vi "LIDAR Sensor Fusion 2.vi"() -> ()   [LabVIEW 2019]
panel:
  in  "Pointed at Target":bool
  out "Fused Range (in)":dbl
  in  "Estimate Range (in)":dbl
  in  "LIDAR Range (in)":dbl
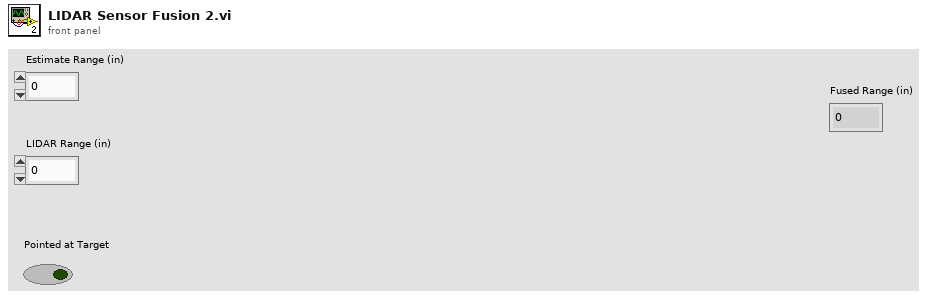
[diagram p1: front panel]
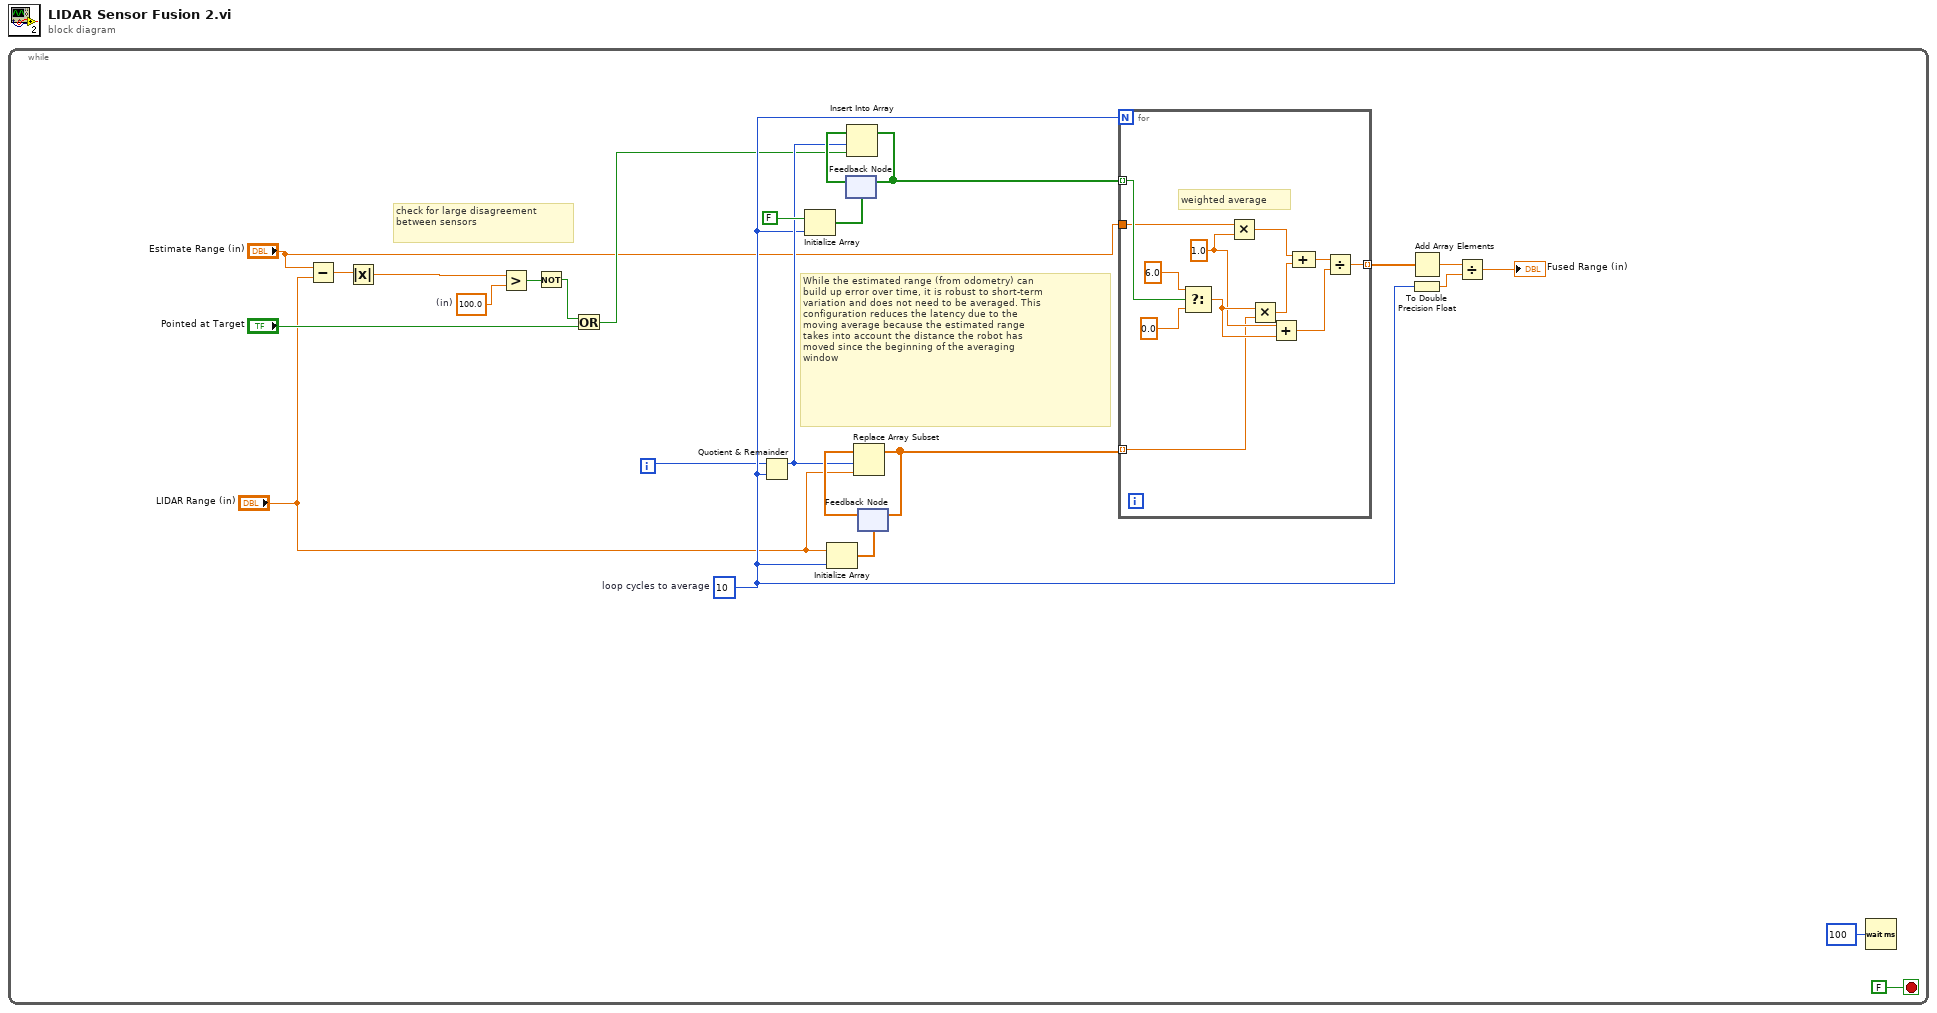
[diagram p0: block diagram]
diagram:
  n1 = while {
    i -> [w2]
    stop <- FALSE stop-if-true
    w6 = 10  # loop cycles to average
    w23 = 100.0  # (in)
    # "While the estimated range (from odometry) can \nbuild up error over time, it is robust to short-term\nvariation and does not need to be averaged. This\nconfiguration reduces the latency due to the \nmoving average because the estimated range\ntakes into account the distance the robot has\nmoved since the beginning of the averaging \nwindow"
    # "check for large disagreement\nbetween sensors"
    n2 = Subtract(x="Estimate Range (in)", y="LIDAR Range (in)") -> (x-y=w25:dbl)
    n3 = Absolute Value(x=w25) -> (abs(x)=w24:dbl)
    n4 = Greater?(x=w24, y=w23) -> (0:w22:bool)
    n5 = Not(x=w22) -> (.not. x?=w21:bool)
    n6 = Or(x=w21, y="Pointed at Target") -> (x .or. y?=w4:bool)
    n7 = Quotient & Remainder(x=w2, y=w6) -> (x-y*floor(x/y)=w10:i32)  [unwired: 1 out]
    n8 = Initialize Array(FALSE, w6) -> (w13:bool[])
    n9 = Initialize Array("LIDAR Range (in)", w6) -> (w17:dbl[])
    n10 = feedback #1(w13) -> (w15:bool[])
    n11 = Insert Into Array(array=w15, index=w10, new element=w4) -> (w12:bool[])
    n12 = feedback-in #1(w12) -> ()
    n13 = feedback #2(w17) -> (w16:dbl[])
    n14 = Replace Array Subset(array=w16, new element="LIDAR Range (in)", index=w10) -> (w11:dbl[])
    n15 = feedback-in #2(w11) -> ()
    n16 = for {
      N: w6 -> [_]
      tunnel: w12 -> [w29] mode=indexing
      tunnel: w11 -> [w28] mode=indexing
      tunnel: "Estimate Range (in)" -> [w27]
      tunnel: [w26] -> w9 mode=indexing
      w30 = 1.0 ("x")
      # "weighted average"
      n17 = Select(t=6.0 ("x"), s=w29, f=0.0) -> (s? t:f=w37:dbl)
      n18 = Multiply(x=w27, y=w30) -> (x*y=w34:dbl)
      n19 = Multiply(x=w37, y=w28) -> (x*y=w35:dbl)
      n20 = Add(x=w30, y=w37) -> (x+y=w36:dbl)
      n21 = Compound Arithmetic op=ADD(w34, w35) -> (w33:dbl)
      n22 = Divide(x=w33, y=w36) -> (x/y=w26:dbl)
    }
    n23 = Add Array Elements(numeric array=w9) -> (sum=w8:dbl)
    n24 = To Double Precision Float(number=w6) -> (double precision float=w7:dbl)
    n25 = Divide(x=w8, y=w7) -> (x/y=→"Fused Range (in)":dbl)
    n26 = Wait (ms)(milliseconds to wait=u32 100) -> ()  [unwired: 1 out]
  }
